vi "LstDevGetSerialNumber.vi"(8 "error in (no error)":errorcluster, 10 "dwId in":u32) -> (0 "error out":errorcluster, 1 "Serial No.":u32, 2 "dwId out":u32)   [LabVIEW 2018, in "LibTiePie.lvlib"]
uses:
  LibTiePie.lvlib
  LabViewHS4/libtiepie.dll
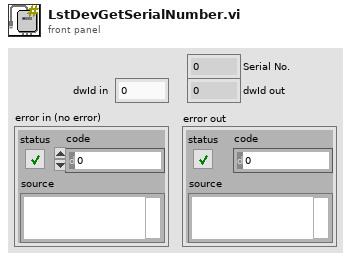
[diagram p1: front panel]
types:
  T1 = enum32{"Reserved1", "Product ID", "Index", "Reserved3", "Serial"}
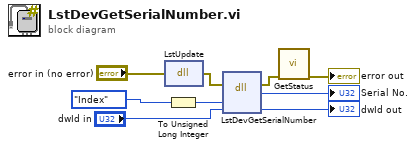
[diagram p0: block diagram]
diagram:
  n1 = dll-call lib="C:/Users/cwaha/Documents/LabViewHS4/libtiepie.dll" fn="LstUpdate"(error in="error in (no error)") -> (error out=w6:errorcluster)  [unwired: 3 in, 1 out]
  n2 = To Unsigned Long Integer(number=T1."Index" ("Indentifier")) -> (unsigned 32bit integer=w7:u32)
  n3 = dll-call lib="C:/Users/cwaha/Documents/LabViewHS4/libtiepie.dll" fn="LstDevGetSerialNumber"(error in=w6, "arg2"=w7, "arg3"="dwId in") -> (error out=w3:errorcluster, "return type"=→"Serial No.":u32, "arg3"=→"dwId out":u32)  [unwired: 3 in, 1 out]
  n4 = call "GetStatus.vi"("error in (no error)"=w3) -> ("error out"=→"error out":errorcluster)  [unwired: 10 in]
